vi "SetImageDisplayType.vi"(8 "Error In":errorcluster, 11 "Value":T1) -> (0 "Error Out":errorcluster, 3 "Palette:Palette Type":u32)   [LabVIEW 2019]
uses:
  Controls/UI_Process_Type.ctl
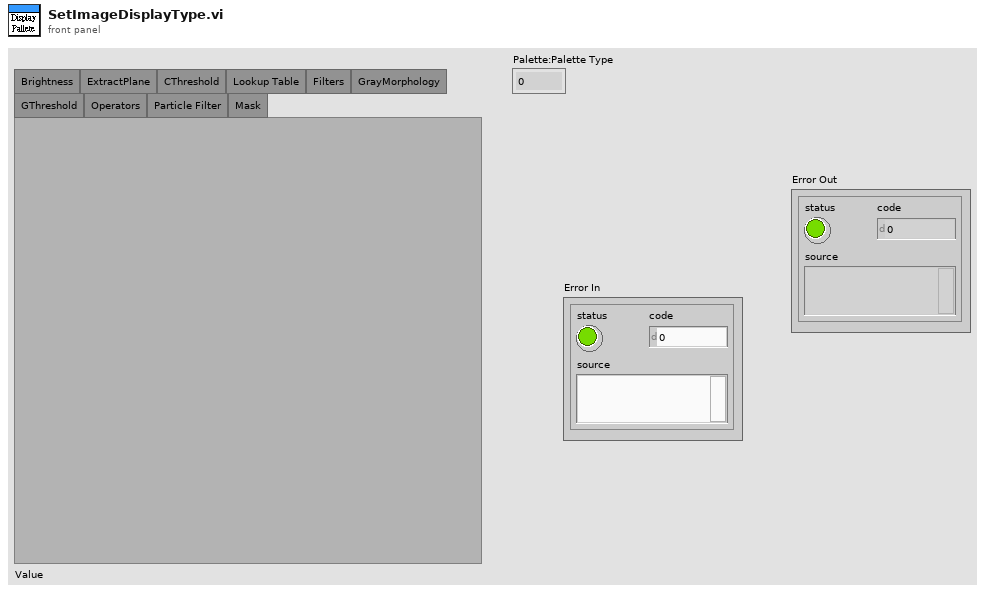
[diagram p1: front panel]
types:
  T1 = typedef "UI_Process_Type.ctl" = enum32{"None", "Brightness", "ExtractPlane", "CThreshold", "Lookup Table", "Filters", "GrayMorphology", "GThreshold", "Operators", "Particle Filter", "Mask"}
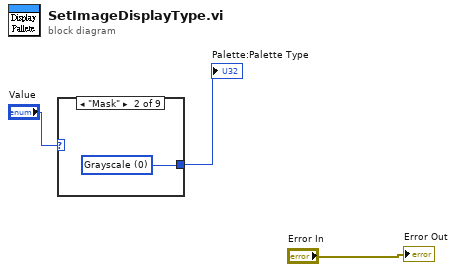
[diagram p0: block diagram]
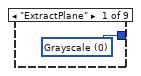
[diagram p2: hidden frame]
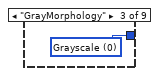
[diagram p3: hidden frame]
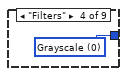
[diagram p4: hidden frame]
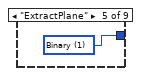
[diagram p5: hidden frame]
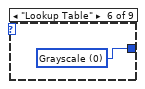
[diagram p6: hidden frame]
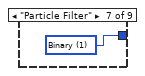
[diagram p7: hidden frame]
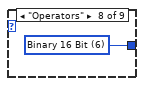
[diagram p8: hidden frame]
diagram:
  n1 = case shown="\"Mask\"" "Value" {
    tunnel: [w4 w5 w6 w7 w8 w9 w10 w11 _] -> w2
    frame "ExtractPlane" {
      w4 = u32 0 items=["Grayscale", "Binary", "Gradient", "Rainbow", "Temperature", "User Defined", "Binary 16 Bit", "Gradient 16 Bit", "Rainbow 16 Bit", "Temperature 16 Bit", "User Defined 16 Bit"] ("Palette:Palette Type")
    }
    frame "Mask" {
      w5 = u32 0 items=["Grayscale", "Binary", "Gradient", "Rainbow", "Temperature", "User Defined", "Binary 16 Bit", "Gradient 16 Bit", "Rainbow 16 Bit", "Temperature 16 Bit", "User Defined 16 Bit"] ("Palette:Palette Type")
    }
    frame "GrayMorphology" {
      w6 = u32 0 items=["Grayscale", "Binary", "Gradient", "Rainbow", "Temperature", "User Defined", "Binary 16 Bit", "Gradient 16 Bit", "Rainbow 16 Bit", "Temperature 16 Bit", "User Defined 16 Bit"] ("Palette:Palette Type")
    }
    frame "Filters" {
      w7 = u32 0 items=["Grayscale", "Binary", "Gradient", "Rainbow", "Temperature", "User Defined", "Binary 16 Bit", "Gradient 16 Bit", "Rainbow 16 Bit", "Temperature 16 Bit", "User Defined 16 Bit"] ("Palette:Palette Type")
    }
    frame "ExtractPlane" {
      w8 = u32 1 items=["Grayscale", "Binary", "Gradient", "Rainbow", "Temperature", "User Defined", "Binary 16 Bit", "Gradient 16 Bit", "Rainbow 16 Bit", "Temperature 16 Bit", "User Defined 16 Bit"] ("Palette:Palette Type")
    }
    frame "Lookup Table" {
      w9 = u32 0 items=["Grayscale", "Binary", "Gradient", "Rainbow", "Temperature", "User Defined", "Binary 16 Bit", "Gradient 16 Bit", "Rainbow 16 Bit", "Temperature 16 Bit", "User Defined 16 Bit"] ("Palette:Palette Type")
    }
    frame "Particle Filter" {
      w10 = u32 1 items=["Grayscale", "Binary", "Gradient", "Rainbow", "Temperature", "User Defined", "Binary 16 Bit", "Gradient 16 Bit", "Rainbow 16 Bit", "Temperature 16 Bit", "User Defined 16 Bit"] ("Palette:Palette Type")
    }
    frame "Operators" {
      w11 = u32 6 items=["Grayscale", "Binary", "Gradient", "Rainbow", "Temperature", "User Defined", "Binary 16 Bit", "Gradient 16 Bit", "Rainbow 16 Bit", "Temperature 16 Bit", "User Defined 16 Bit"] ("Palette:Palette Type")
    }
    frame "None", Default {
    }
  }
  "Palette:Palette Type" <- w2
  "Error Out" <- "Error In"
